vi "PDP Channels= Message.vi"(0 "Channel":string[](array[string])) -> ()   [LabVIEW 2009]
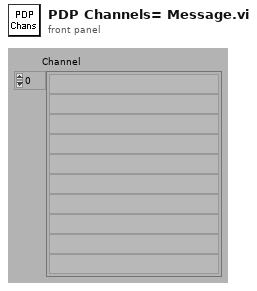
[diagram p1: front panel]
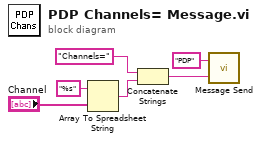
[diagram p0: block diagram]
diagram:
  n1 = Array To Spreadsheet String(array="Channel", 3:"%s" ("format string")) -> (spreadsheet string=w2:string)  [unwired: 1 in]
  n2 = Concatenate Strings("Channels=" ("Substring"), w2) -> (w3:string)
  n3 = call "Message Send.vi"("Message"=w3, "Destination"="PDP") -> ()
